vi "new report subVI.vi"(0 "report in":refnum<class "NI_Excel.lvclass">, 1 "window state (normal)":T1(ring)=enum."normal", 5 "display alerts? (F)":bool, 7 "template (empty)":path, 9 "machine name (empty)":string, 11 "error in (no error)":errorcluster) -> (4 "report out":refnum<class "NI_Excel.lvclass">, 15 "error out":errorcluster)   [LabVIEW 2020, in "NI_Excel.lvclass"]
uses:
  <vilib>/Utility/NIReport.llb/Excel/NI_Excel.lvclass
  <vilib>/Utility/NIReport.llb/Excel/NI_Excel.lvclass/NI_Excel.ctl
  <vilib>/addons/_office/NI_ReportGenerationToolkit.lvlib
  <vilib>/Utility/NIReport.llb/NI_ReportGenerationCore.lvlib
panel:
  in  "Excel._Application":refnum<k7>
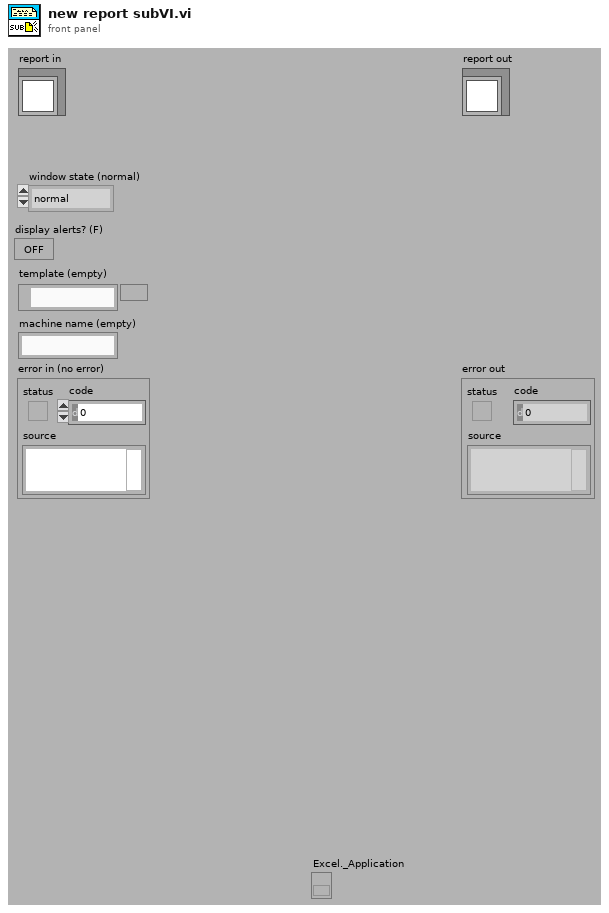
[diagram p1: front panel]
types:
  T1 = enum16{"maximized", "minimized", "normal", "no change"}
  T2 = cluster{"Application":refnum<k7>, "Workbook":refnum<k7>, "Worksheet":refnum<k7>, "Shapes":refnum<k7>, "Worksheets":refnum<k7>}
  T3 = typedef "NI_ReportGenerationCore.lvlib/Report Data Members.ctl" = cluster{"font":T4, "from template?":bool}
  T4 = typedef "NI_ReportGenerationCore.lvlib/font.ctl" = cluster{"font name":string, "font size":dbl, "bold":u16, "italic":u16, "underline":u16, "strike through":u16, "font color":u32}
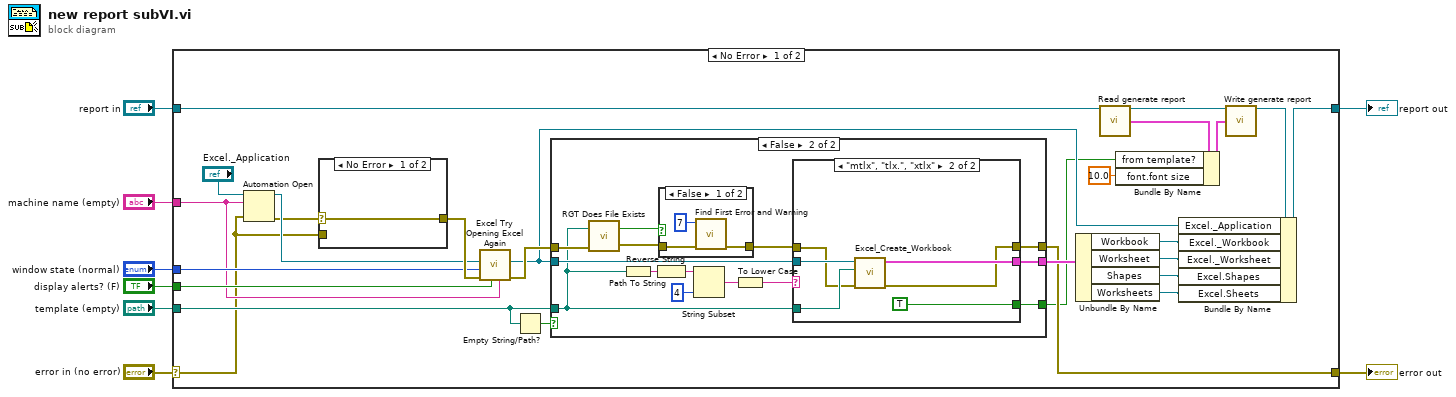
[diagram p0: block diagram]
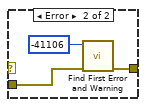
[diagram p2: hidden frame]
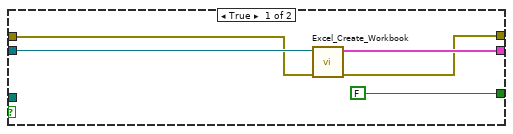
[diagram p3: hidden frame]
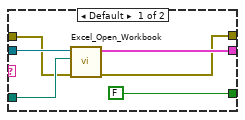
[diagram p5: hidden frame]
diagram:
  n1 = case shown="No Error" "error in (no error)" {
    selector: "error in (no error)" -> [w17 w75]
    tunnel: [w16 w75] -> w7
    tunnel: [w22 w74] -> w5
    tunnel: "report in" -> [w15 w74]
    tunnel: "template (empty)" -> [w21 _]
    tunnel: "window state (normal)" -> [w20 _]
    tunnel: "display alerts? (F)" -> [w19 _]
    tunnel: "machine name (empty)" -> [w18 _]
    frame No Error {
      n2 = Automation Open(machine name=w18, error in (no error)=w17, Automation Refnum="Excel._Application") -> (Automation Refnum=w31:refnum<k7>, error out=w30:errorcluster)  [unwired: 1 out]
      n3 = case shown="No Error" w30 {
        selector: w30 -> [w35 _]
        tunnel: [w35 w37] -> w33
        tunnel: w17 -> [_ w36]
        frame No Error {
        }
        frame Error {
          n4 = call <vilib>:"Find First Error and Warning.vi"("error in (no error)"=w36, "error code"=-41106) -> ("error out"=w37:errorcluster)  [unwired: 5 out]
        }
      }
      n5 = call <vilib>:"Excel Try Opening Excel Again.vi"("machine name (empty)"=w18, "display alerts? (F)"=w19, "error in (no error)"=w33, "window state (normal)"=w20, "Excel._Application in"=w31) -> ("error out"=w34:errorcluster, "Excel._Application out"=w32:refnum<k7>)  [unwired: 1 in, 4 out]
      n6 = Empty String/Path?(string/path=w21) -> (empty?=w28:bool)
      n7 = case shown="False" w28 {
        tunnel: w32 -> [w42 w56]
        tunnel: w34 -> [w41 w51]
        tunnel: [w39 w57] -> w16
        tunnel: w21 -> [_ w48]
        tunnel: [w40 w55] -> w27
        tunnel: [FALSE w46] -> w9
        frame True {
          n8 = call <vilib>:"Excel_Create_Workbook.vi"("error in (no error)"=w41, "excel application"=w42) -> ("error out"=w39:errorcluster, "references"=w40:T2)  [unwired: 1 in, 7 out]
        }
        frame False {
          n9 = call <vilib>:"RGT Does File Exists.vi"("error in (no error)"=w51, "path"=w48) -> ("error out"=w50:errorcluster, "file exists?"=w47:bool)
          n10 = Path To String(path=w48) -> (string=w54:string)
          n11 = Reverse String(1:w54) -> (0:w53:string)
          n12 = case shown="False" w47 {
            tunnel: w50 -> [w60 w61]
            tunnel: [w58 w61] -> w49
            frame False {
              n13 = call <vilib>:"Find First Error and Warning.vi"("error in (no error)"=w60, "error code"=7) -> ("error out"=w58:errorcluster)  [unwired: 5 out]
            }
            frame True {
            }
          }
          n14 = String Subset(string=w53, length (rest)=4 ("length (rest)")) -> (substring=w45:string)  [unwired: 1 out]
          n15 = To Lower Case(string=w45) -> (all lower case string=w44:string)
          n16 = case shown="\"mtlx\", \"tlx.\", \"xtlx\"" w44 {
            tunnel: w49 -> [w62 w68]
            tunnel: [w63 w69] -> w57
            tunnel: w56 -> [w65 w72]
            tunnel: w48 -> [w66 w71]
            tunnel: [w64 w70] -> w55
            tunnel: [FALSE TRUE] -> w46
            frame Default {
              n17 = call <vilib>:"Excel_Open_Workbook.vi"("error in (no error)"=w62, "worksheet path"=w66, "excel application"=w65) -> ("error out"=w63:errorcluster, "references"=w64:T2)  [unwired: 7 out]
            }
            frame "mtlx", "tlx.", "xtlx" {
              n18 = call <vilib>:"Excel_Create_Workbook.vi"("error in (no error)"=w68, "Path"=w71, "excel application"=w72) -> ("error out"=w69:errorcluster, "references"=w70:T2)  [unwired: 7 out]
            }
          }
        }
      }
      n19 = Unbundle By Name(w27) -> ("Workbook"=w23:refnum<k7>, "Worksheet"=w24:refnum<k7>, "Shapes"=w25:refnum<k7>, "Worksheets"=w26:refnum<k7>)
      n20 = call-dynamic "Read generate report.vi"("report in"=w15) -> ("report out"=w14:refnum<class "NI_Excel.lvclass">, "generate report"=w12:T3)  [unwired: 12 in, 1 out]
      n21 = Bundle By Name(cluster=w12, "from template?"=w9, "font.font size"=10.0) -> (w11:T3)
      n22 = call-dynamic "Write generate report.vi"("report in"=w14, "generate report"=w11) -> ("report out"=w13:refnum<class "NI_Excel.lvclass">)  [unwired: 12 in, 1 out]
      n23 = Bundle By Name(cluster=w13, "Excel._Application"=w32, "Excel._Workbook"=w23, "Excel._Worksheet"=w24, "Excel.Shapes"=w25, "Excel.Sheets"=w26) -> (w22:refnum<class "NI_Excel.lvclass">)
    }
    frame Error {
    }
  }
  "error out" <- w7
  "report out" <- w5
